vi "MRC String to LV String.vi"(11 "MRC String":T1) -> (3 "LV String":string)   [LabVIEW 2026, in "MrcLib.lvlib"]
uses:
  MrcLib.lvlib
  FRC_NetworkTablesLV.so
  Types/MRC String.ctl
panel:
  in  "String":string
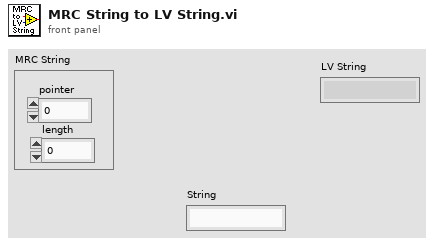
[diagram p1: front panel]
types:
  T1 = typedef "MRC String.ctl" = cluster{"pointer":u64, "length":u64}
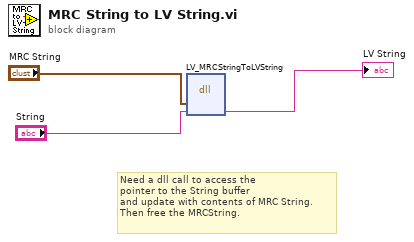
[diagram p0: block diagram]
diagram:
  # "Need a dll call to access the\npointer to the String buffer\nand update with contents of MRC String.\nThen free the MRCString."
  n1 = dll-call lib="FRC_NetworkTablesLV.*" fn="LV_MRCStringToLVString"("mrcstr"="MRC String", "lvstr"="String") -> ("lvstr"=→"LV String":string)  [unwired: 5 in, 2 out]
